vi "gamepad to velocity.vi"(6 "max 3 axis":dbl, 8 "max 2 axis":dbl, 9 "max 1 axis":dbl, 10 "joystick sub":dbl, 11 "joystick main":dbl) -> (1 "lower bound":dbl, 2 "upper bound":dbl, 3 "Velocity":dbl)   [LabVIEW 2012]
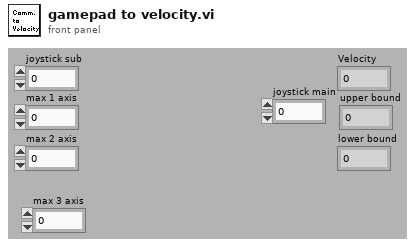
[diagram p1: front panel]
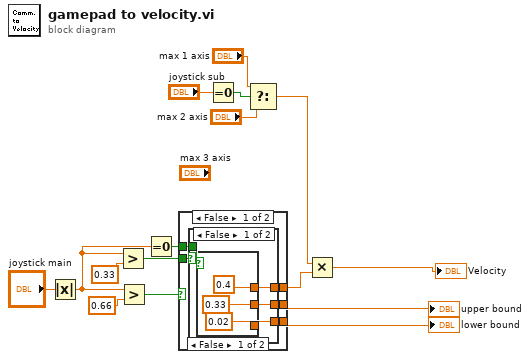
[diagram p0: block diagram]
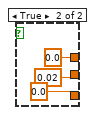
[diagram p2: hidden frame]
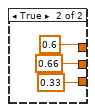
[diagram p3: hidden frame]
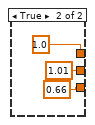
[diagram p4: hidden frame]
diagram:
  n1 = Absolute Value(x="joystick main") -> (abs(x)=w2:dbl)
  n2 = Greater?(x=w2, y=0.33) -> (0:w14:bool)
  n3 = Greater?(x=w2, y=0.66 ("Numeric")) -> (0:w16:bool)
  n4 = Equal To 0?(x=w2) -> (x = 0?=w1:bool)
  n5 = case shown="False" w16 {
    tunnel: w14 -> [w21 _]
    tunnel: [w20 1.0 ("y")] -> w12
    tunnel: [w19 1.01 ("y")] -> w4
    tunnel: [w18 0.66 ("y")] -> w3
    tunnel: w1 -> [w17 _]
    frame False {
      n6 = case shown="False" w21 {
        tunnel: [w23 0.6 ("y")] -> w20
        tunnel: [w24 0.66 ("y")] -> w19
        tunnel: [w25 0.33 ("y")] -> w18
        tunnel: w17 -> [w22 _]
        frame False {
          n7 = case shown="False" w22 {
            tunnel: [0.02 ("y") 0.0 ("y")] -> w25
            tunnel: [0.33 ("y") 0.02 ("y")] -> w24
            tunnel: [0.4 ("y") 0.0 ("y")] -> w23
            frame False {
            }
            frame True {
            }
          }
        }
        frame True {
        }
      }
    }
    frame True {
    }
  }
  "upper bound" <- w4
  "lower bound" <- w3
  n8 = Equal To 0?(x="joystick sub") -> (x = 0?=w9:bool)
  n9 = Select(t="max 1 axis", s=w9, f="max 2 axis") -> (s? t:f=w5:dbl)
  n10 = Multiply(x=w5, y=w12) -> (x*y=→"Velocity":dbl)
